vi "Lab2a.vi"() -> ()   [LabVIEW 2015]
panel:
  out "Number of iterations":u32
  out "Current number":u32
  in  "Number to match":u32 max=1000 step=1
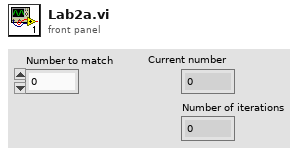
[diagram p1: front panel]
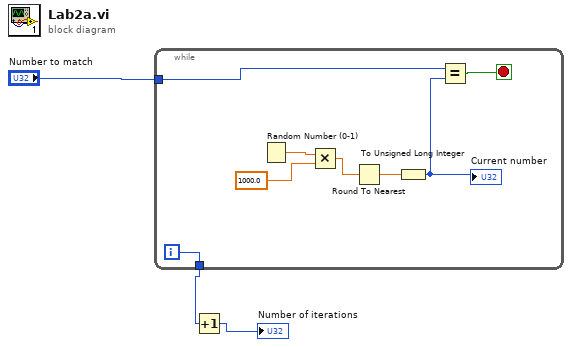
[diagram p0: block diagram]
diagram:
  n1 = while {
    tunnel: "Number to match" -> [w5]
    tunnel: [w4] -> w1
    i -> [w4]
    stop <- w9 stop-if-true
    n2 = Random Number (0-1)() -> (number: 0 to 1=w11:dbl)
    n3 = Multiply(x=w11, y=1000.0) -> (x*y=w10:dbl)
    n4 = Round To Nearest(number=w10) -> (nearest integer value=w7:dbl)
    n5 = To Unsigned Long Integer(number=w7) -> (unsigned 32bit integer=w6:u32)
    "Current number" <- w6
    n6 = Equal?(x=w5, y=w6) -> (x = y?=w9:bool)
  }
  n7 = Increment(x=w1) -> (x+1=→"Number of iterations":i32)
